vi "Simulator.vi"() -> ()   [LabVIEW 2019]
uses:
  <vilib>/Utility/file.llb/Read Delimited Spreadsheet (string).vi
panel:
  out "Progress":dbl(slide) scale=0.0..1.0
  out "Intake State":string
  out "CTRE":cluster{"String":dbl, "String":dbl}(graph)
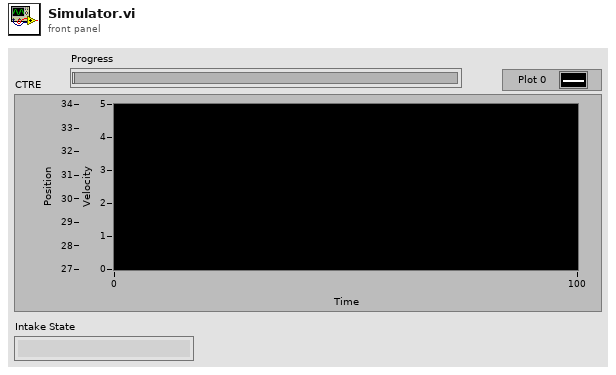
[diagram p1: front panel]
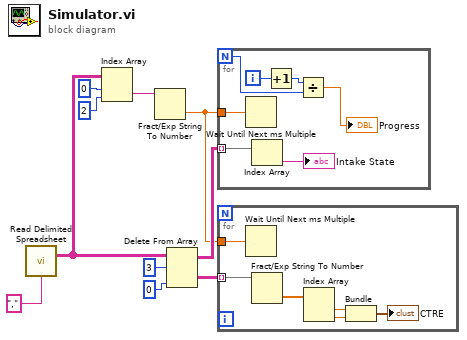
[diagram p0: block diagram]
diagram:
  n1 = call-poly <vilib>:"Read Delimited Spreadsheet.vi"("delimiter (\\t)"="," ("delimiter (\\t)")) -> ("all rows"=w2:string[][])  [unwired: 9 in, 5 out]
  n2 = Index Array(array=w2, index (row)=0, index (col)=2 ("disabled index (col)")) -> (element=w4:string)
  n3 = Fract/Exp String To Number(string=w4) -> (number=w3:dbl)  [unwired: 3 in, 1 out]
  n4 = Delete From Array(array=w2, length=3, index (col)=0 ("disabled index (col)")) -> (deleted portion=w8:string[][], array with subset deleted=w7:string[][])  [unwired: 1 in]
  n5 = for {
    N -> [w14]
    tunnel: w7 -> [w16] mode=indexing
    tunnel: w3 -> [w17]
    i -> [w13]
    n6 = Wait Until Next ms Multiple(millisecond multiple=w17) -> ()  [unwired: 1 out]
    n7 = Index Array(array=w16) -> (element=→"Intake State":string)  [unwired: 1 in]
    n8 = Increment(x=w13) -> (x+1=w12:i32)
    n9 = Divide(x=w12, y=w14) -> (x/y=→"Progress":dbl)
  }
  n10 = for {
    tunnel: w8 -> [w23] mode=indexing
    tunnel: w3 -> [w18]
    n11 = Wait Until Next ms Multiple(millisecond multiple=w18) -> ()  [unwired: 1 out]
    n12 = Fract/Exp String To Number(string=w23) -> (number=w19:dbl[])  [unwired: 3 in, 1 out]
    n13 = Index Array(array=w19) -> (element #1=w22:dbl, element #2=w21:dbl)  [unwired: 2 in]
    n14 = Bundle("String"=w22, "String"=w21) -> (→"CTRE":cluster{"String":dbl, "String":dbl})  [unwired: 1 in]
  }
